vi "Property_Tree Tag_Decode2.vi"(11 "Tag In":string) -> (3 "TagData":T1)   [LabVIEW 2023]
doc: "Decode from tree tag the unique ID string for a method or property, and return the short and long names. The long name is the colon-dlimited name as it appears in the property node. The short name is the value afte the colon, eg:\n\nLong = Bounds:Legnth\nShort = Legnth\nParent= Bounds"
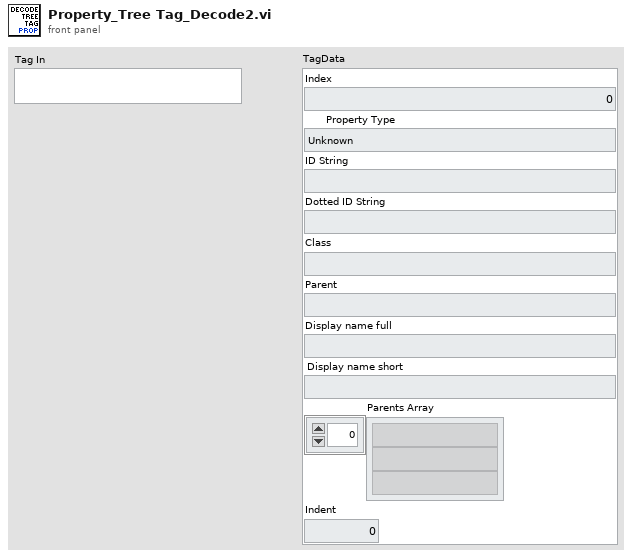
[diagram p1: front panel]
types:
  T1 = cluster{"Index":u16, "Property Type":enum16{"Unknown", "Base", "Scripting", "Private", "Deprecated", "None", "Divider"}, "ID String":string, "Dotted ID String":string, "Class":string, "Parent":string, "Display name full":string, "Display name short":string, "Parents Array":string[], "Indent":u16}
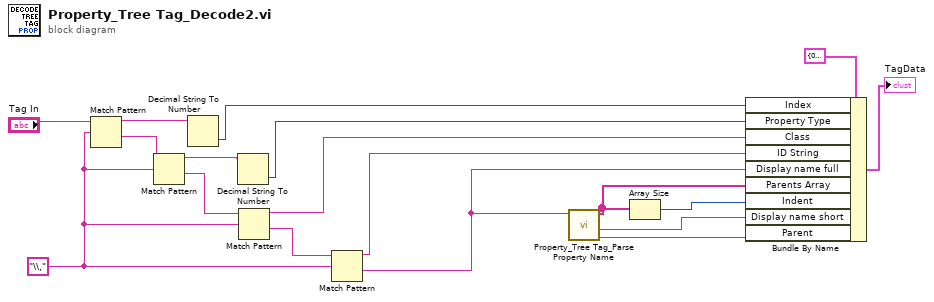
[diagram p0: block diagram]
diagram:
  w13 = "\\," ("search string")
  n1 = Match Pattern(string="Tag In", regular expression=w13) -> (before substring=w17:string, after substring=w16:string)  [unwired: 1 in, 2 out]
  n2 = Match Pattern(string=w16, regular expression=w13) -> (before substring=w14:string, after substring=w15:string)  [unwired: 1 in, 2 out]
  n3 = Decimal String To Number(string=w17) -> (number=w11:i32)  [unwired: 2 in, 1 out]
  n4 = Decimal String To Number(string=w14) -> (number=w10:i32)  [unwired: 2 in, 1 out]
  n5 = Match Pattern(string=w15, regular expression=w13) -> (before substring=w9:string, after substring=w12:string)  [unwired: 1 in, 2 out]
  n6 = Match Pattern(string=w12, regular expression=w13) -> (before substring=w8:string, after substring=w4:string)  [unwired: 1 in, 2 out]
  n7 = call "Property_Tree Tag_Parse Property Name.vi"("Tag Property Name"=w4) -> ("Parent"=w1:string, "Display name short"=w3:string, "Parent Array"=w2:string[])  [unwired: 7 in, 1 out]
  n8 = Array Size(array=w2) -> (size(s)=w6:i32)
  n9 = Bundle By Name(cluster=T1 {"Index"=0, "Property Type"=enum."Unknown", "ID String"="", "Dotted ID String"="", "Class"="", "Parent"="", "Display name full"="", "Display name short"="", "Parents Array"=[], "Indent"=0} ("TagData"), "Index"=w11, "Property Type"=w10, "Class"=w9, "ID String"=w8, "Display name full"=w4, "Parents Array"=w2, "Indent"=w6, "Display name short"=w3, "Parent"=w1) -> (→"TagData":T1)
